vi "open configuration file.vi"(8 "error in (no error)":errorcluster, 11 "Configuration File in":refnum<class "Configuration File.lvclass">) -> (0 "error out":errorcluster, 3 "Configuration File out":refnum<class "Configuration File.lvclass">)   [LabVIEW 2018, in "Configuration File.lvclass"]
uses:
  Configuration File.lvclass
  Configuration File.lvclass/Configuration File.ctl
  <vilib>/Utility/config.llb/NI_LVConfig.lvlib
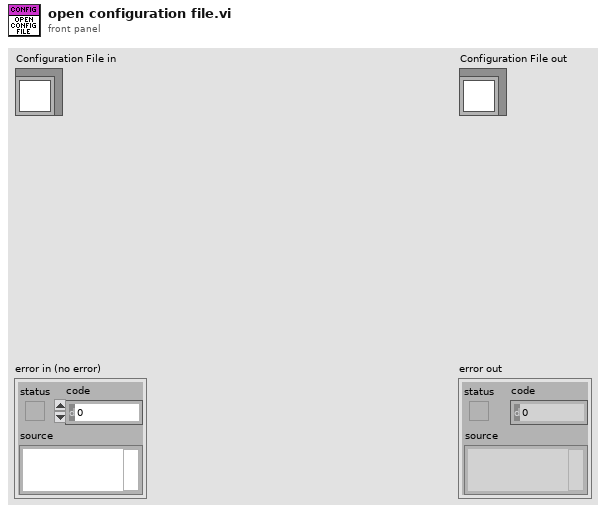
[diagram p1: front panel]
types:
  T1 = typedef "NI_LVConfig.lvlib/Config Data RefNum.ctl" = refnum<k1>
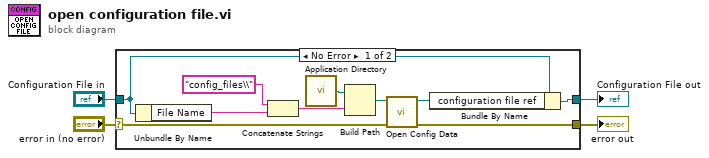
[diagram p0: block diagram]
diagram:
  n1 = case shown="No Error" "error in (no error)" {
    selector: "error in (no error)" -> [w14 w16]
    tunnel: [w13 w16] -> w3
    tunnel: [w12 w15] -> w1
    tunnel: "Configuration File in" -> [w10 w15]
    frame No Error {
      n2 = Unbundle By Name(w10) -> ("File Name"=w7:string)
      n3 = Concatenate Strings("config_files\\", w7) -> (w8:string)
      n4 = call <vilib>:"Application Directory.vi"() -> ("Application Directory"=w9:path)
      n5 = Build Path(base path=w9, name or relative path=w8) -> (appended path=w5:path)
      n6 = call <vilib>:"Open Config Data.vi"("error in (no error)"=w14, "configuration file path"=w5) -> ("error out"=w13:errorcluster, "refnum"=w11:T1)  [unwired: 7 in, 1 out]
      n7 = Bundle By Name(cluster=w10, "configuration file ref"=w11) -> (w12:refnum<class "Configuration File.lvclass">)
    }
    frame Error {
    }
  }
  "error out" <- w3
  "Configuration File out" <- w1
